vi "Return Available Buffer.vi"(8 "error in (no error)":errorcluster, 10 "DMA Memory":refnum<data-value>, 11 "RFSA DAQ in":refnum<class "RFSA DAQ.lvclass">) -> (0 "error out":errorcluster, 3 "RFSA DAQ out":refnum<class "RFSA DAQ.lvclass">)   [LabVIEW 2025, in "RFSA DAQ.lvlib" / "RFSA DAQ.lvclass"]
uses:
  RFSA DAQ.lvclass
  RFSA DAQ.lvclass/RFSA DAQ.ctl
  DAQ Interface/DAQ Interface/DAQ Interface.lvclass
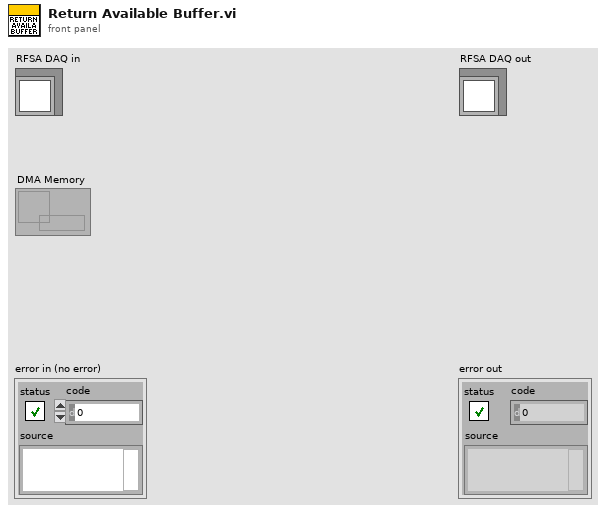
[diagram p1: front panel]
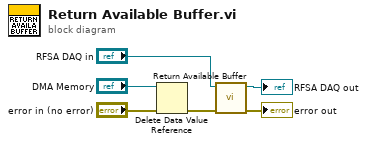
[diagram p0: block diagram]
diagram:
  n1 = Delete Data Value Reference(data value reference="DMA Memory", error in="error in (no error)") -> (error out=w1:errorcluster)  [unwired: 1 out]
  n2 = call-parent "Return Available Buffer.vi"("error in (no error)"=w1, "DAQ Interface in"="RFSA DAQ in") -> ("error out"=→"error out":errorcluster, "DAQ Interface out"=→"RFSA DAQ out":refnum<class "RFSA DAQ.lvclass">)  [unwired: 8 in]
